vi "ObtainSingletonRef.vi"(8 "error in (no error)":errorcluster) -> (0 "error out":errorcluster, 3 "data value reference":refnum<data-value>)   [LabVIEW 2017, in "TimerEngine.lvlib" / "TimerEngine.lvclass"]
uses:
  TimerEngine.lvclass
  _Typedef/WatchDogData--Cluster.ctl
  _Typedef/Timer-UserEvent.ctl
  TimerEngine.lvclass/TimerEngine.ctl
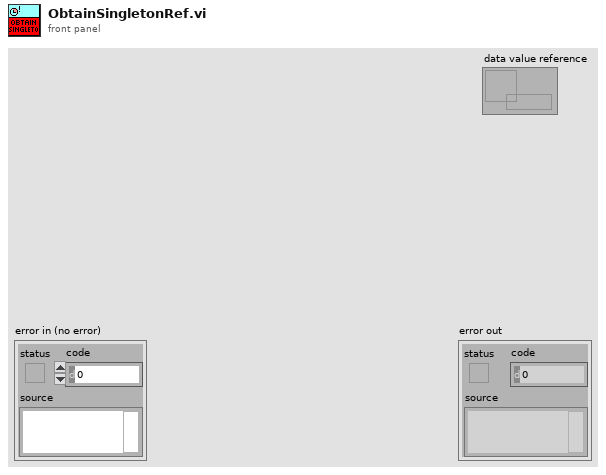
[diagram p1: front panel]
types:
  T1 = typedef "TimerEngine.lvlib/TimerEngine.lvclass/WatchDogData--Cluster.ctl" = cluster{"TimePeroid(ms)":i32, "ResponeQueue":refnum<queue>, "TimerEngineState":refnum<class>}
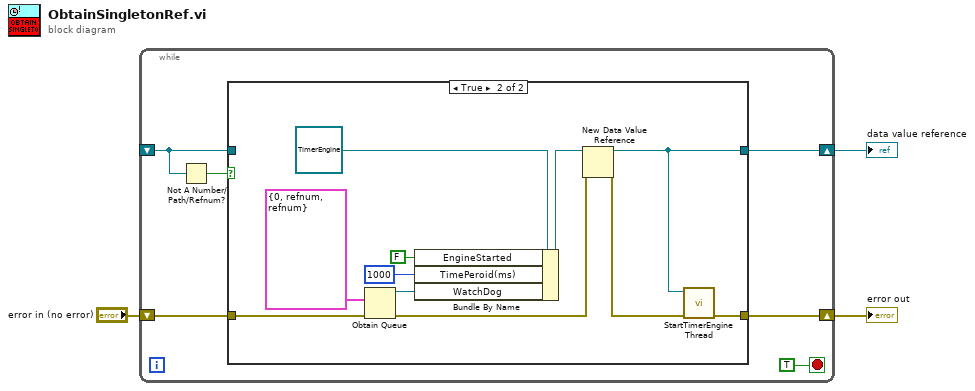
[diagram p0: block diagram]
diagram:
  n1 = while {
    shift-right: [w8] -> w2
    shift-left: "error in (no error)" -> [w9]
    shift-right: [w7] -> w1
    shift-left: _ -> [w4]
    stop <- TRUE stop-if-true
    n2 = Not A Number/Path/Refnum?(number/path/refnum=w4) -> (NaN/Path/Refnum?=w5:bool)
    n3 = case shown="True" w5 {
      tunnel: w9 -> [w10 w21]
      tunnel: [w10 w15] -> w8
      tunnel: [w11 w12] -> w7
      tunnel: w4 -> [w11 _]
      frame False {
      }
      frame True {
        n4 = Obtain Queue(element data type=T1 {"TimePeroid(ms)"=0, "ResponeQueue"=refnum, "TimerEngineState"=refnum} ("Request"), error in (no error)=w21) -> (queue out=w17:refnum<queue>, error out=w19:errorcluster)  [unwired: 3 in, 1 out]
        n5 = Bundle By Name(cluster=refnum<class "TimerEngine.lvclass"> refnum ("UserEventTimer.lvclass"), "EngineStarted"=FALSE, "TimePeroid(ms)"=1000, "WatchDog"=w17) -> (w18:refnum<class "TimerEngine.lvclass">)
        n6 = New Data Value Reference(data value=w18, error in=w19) -> (data value reference=w12:refnum<data-value>, error out=w20:errorcluster)
        n7 = call "StartTimerEngineThread.vi"("error in (no error)"=w20, "DVR"=w12) -> ("error out"=w15:errorcluster)  [unwired: 9 in]
      }
    }
  }
  "error out" <- w2
  "data value reference" <- w1
